vi "Variant To Data - Generic - 2D array.vi"(8 "Error In":errorcluster, 10 "Type code":i32, 11 "Variant":variant) -> (0 "Error Out":errorcluster, 3 "2D array":dbl[][](array[numeric]))   [LabVIEW 2014]
doc: "<B>Copyright</B>: (c) MHWirth 2015. All rights are reserved.\n\nThis SubVI converts variant data of 2D array type to 2D array of doubles. \n\n<B>Note 2</B>: It does not support 2D arrays of <B>strings</B>.\n\n\nSupported shared variable types:\nCode 1. Boolean\nCode 2 to 5. Int8/16/32/64\nCode 6 to 9. UInt8/16/32/64\nCode 10. Double\nCode 11. Single-precision\nCode 12. String\nCode 13-23 - 1D array of above types except string\n\n<B>Error 7001</B>: Unknown Data Type - Type Code Array (Int32) contains -1 indicating an unknown data type."
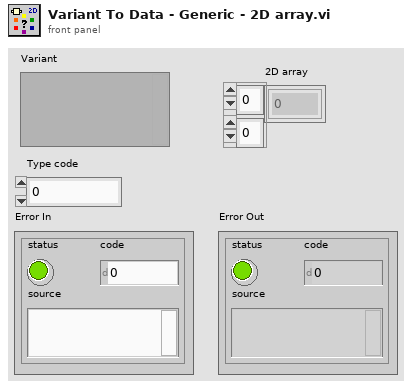
[diagram p1: front panel]
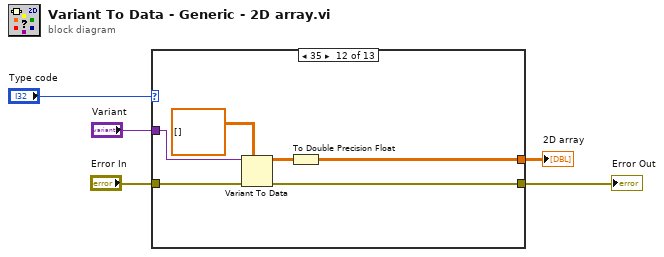
[diagram p0: block diagram]
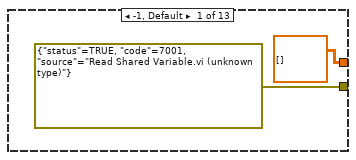
[diagram p2: hidden frame]
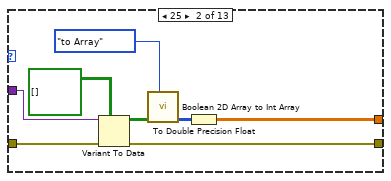
[diagram p3: hidden frame]
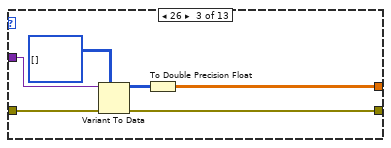
[diagram p4: hidden frame]
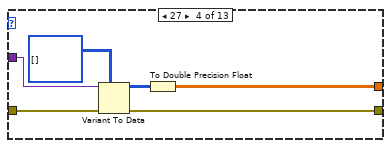
[diagram p5: hidden frame]
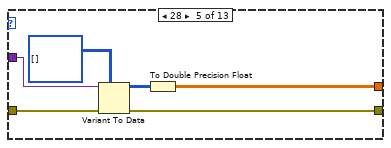
[diagram p6: hidden frame]
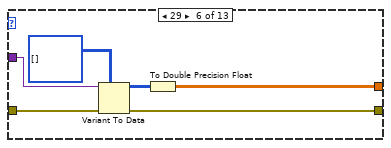
[diagram p7: hidden frame]
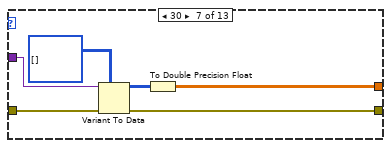
[diagram p8: hidden frame]
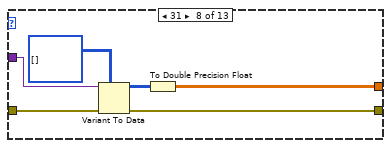
[diagram p9: hidden frame]
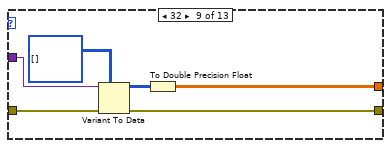
[diagram p10: hidden frame]
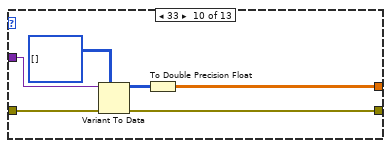
[diagram p11: hidden frame]
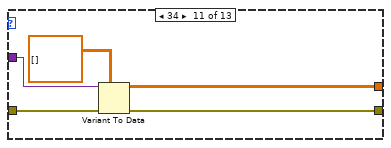
[diagram p12: hidden frame]
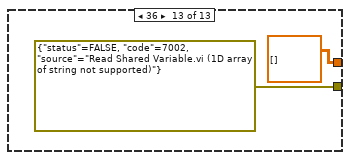
[diagram p13: hidden frame]
diagram:
  n1 = case shown="35" "Type code" {
    tunnel: [errorcluster {"status"=TRUE, "code"=7001, "source"="Read Shared Variable.vi (unknown type)"} ("error constant") w15 w21 w27 w33 w39 w45 w51 w57 w63 w68 w74 errorcluster {"status"=FALSE, "code"=7002, "source"="Read Shared Variable.vi (1D array of string not supported)"} ("Error In")] -> w4
    tunnel: "Error In" -> [_ w14 w20 w26 w32 w38 w44 w50 w56 w62 w67 w73 _]
    tunnel: [dbl[][] [] w11 w16 w22 w28 w34 w40 w46 w52 w58 w64 w69 dbl[][] []] -> w1
    tunnel: "Variant" -> [_ w12 w17 w23 w29 w35 w41 w47 w53 w59 w65 w70 _]
    frame -1, Default {
    }
    frame 25 {
      n2 = Variant To Data(error in=w14, type=bool[][] [], Variant=w12) -> (data=w10:bool[][], error out=w15:errorcluster)
      n3 = call "Boolean 2D Array to Int Array.vi"("Mode"=enum16{"to Array", "to Number"}."to Array" ("Enum"), "Array of Boolean"=w10) -> ("Array out"=w9:u32[][])  [unwired: 8 in]
      n4 = To Double Precision Float(number=w9) -> (double precision float=w11:dbl[][])
    }
    frame 26 {
      n5 = Variant To Data(error in=w20, type=i8[][] [], Variant=w17) -> (data=w19:i8[][], error out=w21:errorcluster)
      n6 = To Double Precision Float(number=w19) -> (double precision float=w16:dbl[][])
    }
    frame 27 {
      n7 = Variant To Data(error in=w26, type=i16[][] [], Variant=w23) -> (data=w25:i16[][], error out=w27:errorcluster)
      n8 = To Double Precision Float(number=w25) -> (double precision float=w22:dbl[][])
    }
    frame 28 {
      n9 = Variant To Data(error in=w32, type=i32[][] [], Variant=w29) -> (data=w31:i32[][], error out=w33:errorcluster)
      n10 = To Double Precision Float(number=w31) -> (double precision float=w28:dbl[][])
    }
    frame 29 {
      n11 = Variant To Data(error in=w38, type=i64[][] [], Variant=w35) -> (data=w37:i64[][], error out=w39:errorcluster)
      n12 = To Double Precision Float(number=w37) -> (double precision float=w34:dbl[][])
    }
    frame 30 {
      n13 = Variant To Data(error in=w44, type=u8[][] [], Variant=w41) -> (data=w43:u8[][], error out=w45:errorcluster)
      n14 = To Double Precision Float(number=w43) -> (double precision float=w40:dbl[][])
    }
    frame 31 {
      n15 = Variant To Data(error in=w50, type=u16[][] [], Variant=w47) -> (data=w49:u16[][], error out=w51:errorcluster)
      n16 = To Double Precision Float(number=w49) -> (double precision float=w46:dbl[][])
    }
    frame 32 {
      n17 = Variant To Data(error in=w56, type=u32[][] [], Variant=w53) -> (data=w55:u32[][], error out=w57:errorcluster)
      n18 = To Double Precision Float(number=w55) -> (double precision float=w52:dbl[][])
    }
    frame 33 {
      n19 = Variant To Data(error in=w62, type=u64[][] [], Variant=w59) -> (data=w61:u64[][], error out=w63:errorcluster)
      n20 = To Double Precision Float(number=w61) -> (double precision float=w58:dbl[][])
    }
    frame 34 {
      n21 = Variant To Data(error in=w67, type=dbl[][] [], Variant=w65) -> (data=w64:dbl[][], error out=w68:errorcluster)
    }
    frame 35 {
      n22 = Variant To Data(error in=w73, type=sgl[][] [], Variant=w70) -> (data=w72:sgl[][], error out=w74:errorcluster)
      n23 = To Double Precision Float(number=w72) -> (double precision float=w69:dbl[][])
    }
    frame 36 {
    }
  }
  "Error Out" <- w4
  "2D array" <- w1
